vi "Query Lock.vi"(8 "error in (no error)":errorcluster, 10 "Motor ID (0)":u8, 11 "VISA resource name":refnum<visa-resource-name>) -> (0 "error out":errorcluster, 2 "EEPROM Locked":bool, 3 "VISA resource name out":refnum<visa-resource-name>)   [LabVIEW 2016, in "Dynamixel Motor.lvlib"]
doc: "Checks to see if the motor has been locked. If it has been locked, then addresses in the EEPROM (0-23) cannot be modified until the motor's power is cycled."
uses:
  Dynamixel Motor.lvlib
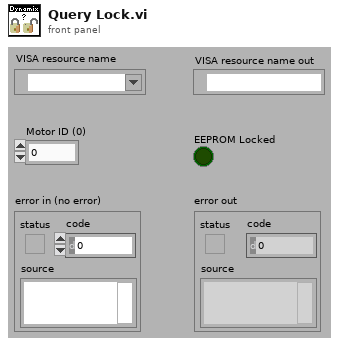
[diagram p1: front panel]
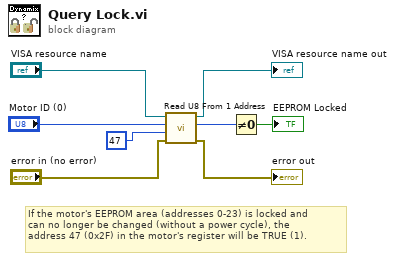
[diagram p0: block diagram]
diagram:
  # "If the motor's EEPROM area (addresses 0-23) is locked and\ncan no longer be changed (without a power cycle), the \naddress 47 (0x2F) in the motor's register will be TRUE (1)."
  n1 = call "Read U8 From 1 Address.vi"("Error in (no error)"="error in (no error)", "Address number (0)"=u8 47 ("Address # DEC"), "Motor ID (0)"="Motor ID (0)", "VISA resource name"="VISA resource name") -> ("error out"=→"error out":errorcluster, "Data"=w4:u8, "VISA resource name out"=→"VISA resource name out":refnum<visa-resource-name>)  [unwired: 5 in]
  n2 = Not Equal To 0?(x=w4) -> (x != 0?=→"EEPROM Locked":bool)
